vi "查看元素在数组中的个数.vi"(8 "字符串":string, 11 "添加的数组":string[](array[string])) -> (0 "大小":i32)   [LabVIEW 2017]
panel:
  out "大小 2":i32
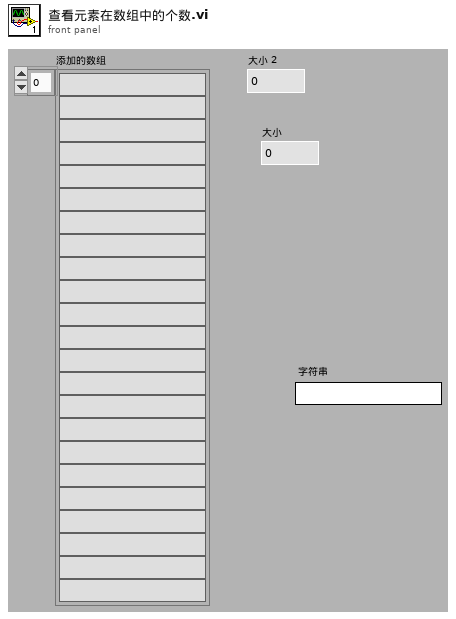
[diagram p1: front panel]
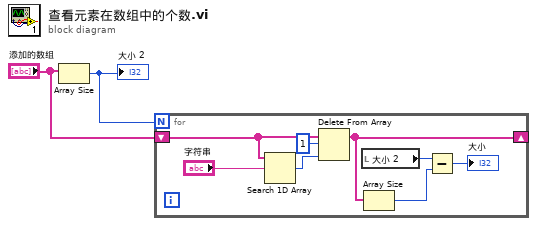
[diagram p0: block diagram]
diagram:
  n1 = Array Size(array="添加的数组") -> (size(s)=w2:i32)
  "大小 2" <- w2
  n2 = for {
    N: w2 -> [_]
    shift-right: [w7] -> _
    shift-left: "添加的数组" -> [w8]
    n3 = Search 1D Array(1D array=w8, element="字符串") -> (index of element=w10:i32)  [unwired: 1 in]
    n4 = Delete From Array(array=w8, length=1 ("长度"), index=w10) -> (array with subset deleted=w7:string[])  [unwired: 1 out]
    n5 = local read "大小 2"() -> (w4:i32)
    n6 = Array Size(array=w7) -> (size(s)=w6:i32)
    n7 = Subtract(x=w4, y=w6) -> (x-y=→"大小":i32)
  }
